vi "test_find_consecutive_close_data.vi"() -> ()   [LabVIEW 2024]
uses:
  <vilib>/Utility/file.llb/Read Delimited Spreadsheet (string).vi
panel:
  out "average":dbl
  in  "csv_data_file_name":string(combo)="low-1.csv"
  in  "python_module_name":string="find_consecutive_close_values.py"
  out "Measures Plot":dbl[][](graph)
  out "data qty":i32
  out "close values":dbl[](array[numeric])
  in  "tolerance%":dbl=4.0 min=0.0 format="%#.4f"
  in  "min_threshold":dbl=10.0 format="%.2f"
  # "Powered by \nPython 3.9.13\n32-bits"
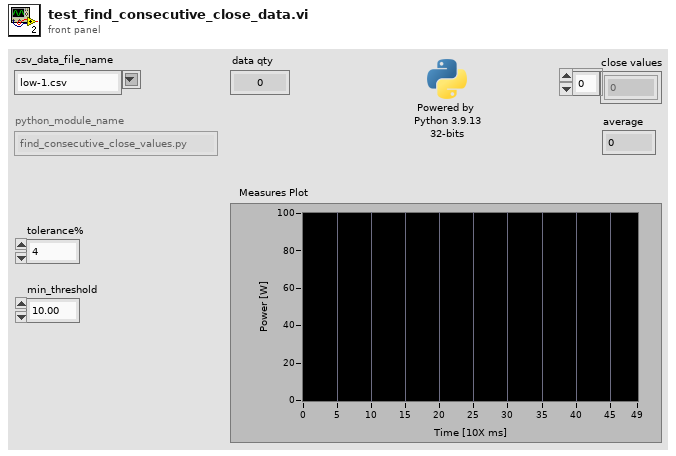
[diagram p1: front panel]
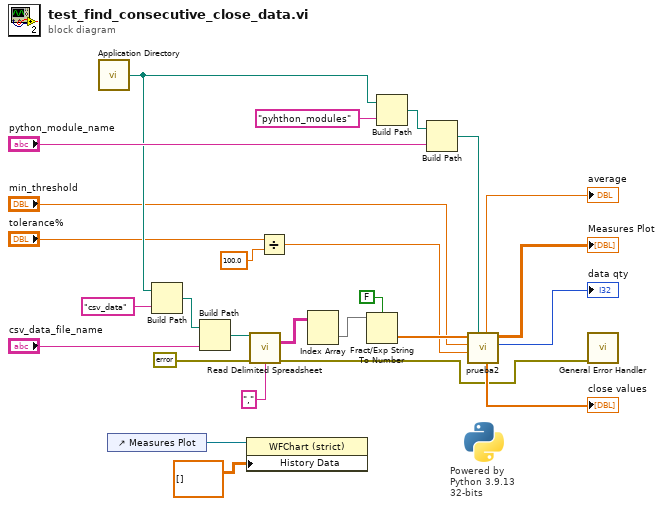
[diagram p0: block diagram]
diagram:
  # "Powered by \nPython 3.9.13\n32-bits"
  n1 = call <vilib>:"Application Directory.vi"() -> ("Application Directory"=w13:path)
  n2 = control-ref of="Measures Plot"() -> (w20:refnum<vi>)
  n3 = Build Path(base path=w13, name or relative path="csv_data") -> (appended path=w16:path)
  n4 = Build Path(base path=w16, name or relative path="csv_data_file_name") -> (appended path=w12:path)
  n5 = property class="WFChart (strict)"(reference=w20, "History Data"=dbl[][] []) -> ()  [unwired: 1 in, 2 out]
  n6 = call-poly <vilib>:"Read Delimited Spreadsheet.vi"("file path (dialog if empty)"=w12, "error in (no error)"=errorcluster {"status"=FALSE, "code"=0, "source"=""} ("error constant"), "delimiter (\\t)"=",") -> ("all rows"=w25:string[][], "error out"=w1:errorcluster)  [unwired: 7 in, 4 out]
  n7 = Divide(x="tolerance%", y=100.0) -> (x/y=w3:dbl)
  n8 = Index Array(array=w25) -> (element=w23:string[])  [unwired: 2 in]
  n9 = Fract/Exp String To Number(use system decimal point (T)=FALSE, string=w23) -> (number=w5:dbl[])  [unwired: 2 in, 1 out]
  n10 = Build Path(base path=w13, name or relative path="pyhthon_modules") -> (appended path=w17:path)
  n11 = Build Path(base path=w17, name or relative path="python_module_name") -> (appended path=w9:path)
  n12 = call "prueba2.vi"("module path"=w9, "tolerance"=w3, "min_threshold"="min_threshold", "data"=w5) -> ("data qty"=→"data qty":i32, "Measures"=→"Measures Plot":dbl[][], "close_values"=→"close values":dbl[], "average"=→"average":dbl)  [unwired: 3 in, 1 out]
  n13 = call <vilib>:"General Error Handler.vi"("error in (no error)"=w1) -> ()  [unwired: 10 in, 5 out]
